vi "Wczytanie_ustawien_DI.vi"(8 "error in (no error)":errorcluster, 10 "Kanały cyfrowe in":refnum<vi>, 11 "Plik konf in":path) -> (0 "error out":errorcluster, 3 "Plik konf out":path)   [LabVIEW 2013]
doc: "Wczytuje ustawienia kontroli DI z pliku\nDI_Konfiguracja.txt"
uses:
  Kontrolki/GUI/DI_aktywacja.ctl
  Kontrolki/GUI/DI_prog.ctl
panel:
  out "output cluster":T1
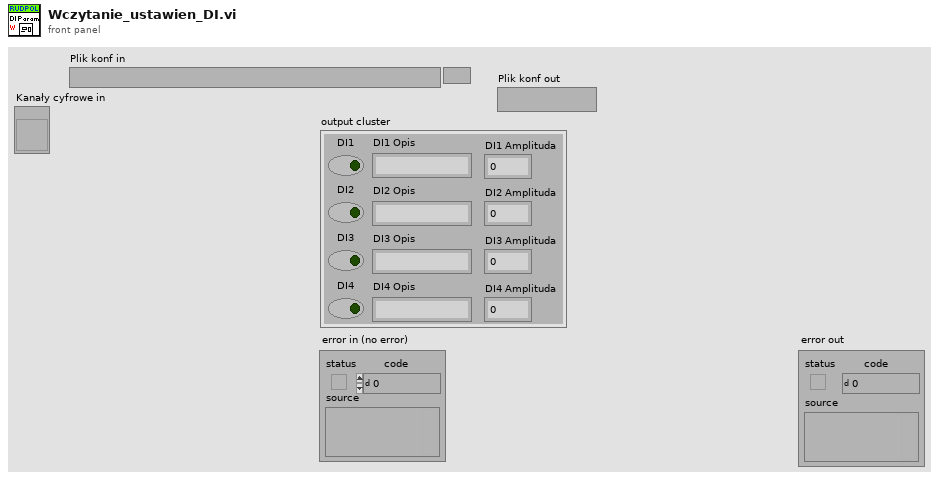
[diagram p1: front panel]
types:
  T1 = typedef "DI_aktywacja.ctl" = cluster{"DI1":bool, "DI2":bool, "DI3":bool, "DI4":bool, "DI1 Opis":string, "DI2 Opis":string, "DI3 Opis":string, "DI4 Opis":string, "DI1 Amplituda":dbl, "DI2 Amplituda":dbl, "DI3 Amplituda":dbl, "DI4 Amplituda":dbl}
  T2 = enum16{"open", "replace", "create", "open or create", "replace or create", "replace or create with confirmation"}
  T3 = typedef "DI_prog.ctl" = enum8{"2,5", "6,0", "12,0"}
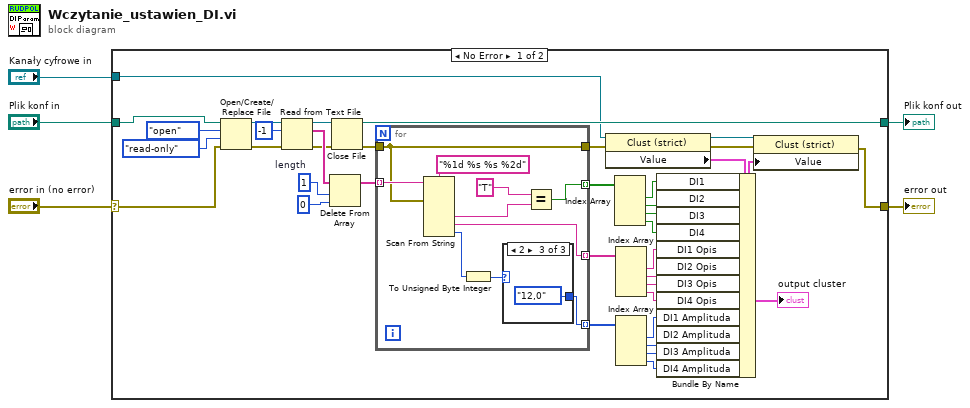
[diagram p0: block diagram]
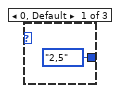
[diagram p2: hidden frame]
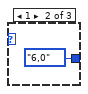
[diagram p3: hidden frame]
diagram:
  n1 = case shown="No Error" "error in (no error)" {
    selector: "error in (no error)" -> [w30 w57]
    tunnel: [w27 w57] -> w4
    tunnel: "Plik konf in" -> [w32 w56]
    tunnel: [w31 w56] -> w2
    tunnel: "Kanały cyfrowe in" -> [w23 _]
    frame No Error {
      w41 = 1  # length
      n2 = Open/Create/Replace File(file path (use dialog)=w32, error in=w30, operation (0:open)=T2."open", access (0:read/write)=enum16{"read/write", "read-only", "write-only"}."read-only") -> (refnum out=w36:refnum<file>, error out=w35:errorcluster)  [unwired: 2 in, 1 out]
      n3 = Read from Text File(file (use dialog)=w36, count=-1, error in=w35) -> (refnum out=w38:refnum<file>, text=w42:string[], error out=w37:errorcluster)  [unwired: 1 in, 1 out]
      n4 = Delete From Array(array=w42, length=w41, index=0) -> (array with subset deleted=w29:string[])  [unwired: 1 out]
      n5 = Close File(refnum=w38, error in=w37) -> (path=w31:path, error out=w28:errorcluster)
      n6 = for {
        tunnel: w29 -> [w51] mode=indexing
        tunnel: w28 -> [w50]
        tunnel: [w50] -> w24
        tunnel: [w47] -> w16 mode=indexing
        tunnel: [w46] -> w15 mode=indexing
        tunnel: [w45] -> w10 mode=indexing
        n7 = Scan From String(format string="%1d %s %s %2d", input string=w51, error in=w50) -> (output 2=w48:string, output 3=w46:string, output 4=w43:i32)  [unwired: 6 in, 3 out]
        n8 = To Unsigned Byte Integer(number=w43) -> (unsigned 8bit integer=w44:u8)
        n9 = case shown="2" w44 {
          tunnel: [DI_prog."2,5" ("DI1 Prog") DI_prog."6,0" ("DI1 Prog") DI_prog."12,0" ("DI1 Prog")] -> w45
          frame 0, Default {
          }
          frame 1 {
          }
          frame 2 {
          }
        }
        n10 = Equal?(x="T" ("y"), y=w48) -> (x = y?=w47:bool)
      }
      n11 = property class="Clust (strict)"(reference=w23, error in=w24) -> (reference out=w26:refnum<vi>, error out=w25:errorcluster, "Value"=w22:T1)
      n12 = Index Array(array=w16) -> (element #1=w20:bool, element #2=w19:bool, element #3=w18:bool, element #4=w17:bool)  [unwired: 4 in]
      n13 = Index Array(array=w15) -> (element #1=w14:string, element #2=w13:string, element #3=w12:string, element #4=w11:string)  [unwired: 4 in]
      n14 = Index Array(array=w10) -> (element #1=w9:T3, element #2=w8:T3, element #3=w7:T3, element #4=w6:T3)  [unwired: 4 in]
      n15 = Bundle By Name(cluster=w22, "DI1"=w20, "DI2"=w19, "DI3"=w18, "DI4"=w17, "DI1 Opis"=w14, "DI2 Opis"=w13, "DI3 Opis"=w12, "DI4 Opis"=w11, "DI1 Amplituda"=w9, "DI2 Amplituda"=w8, "DI3 Amplituda"=w7, "DI4 Amplituda"=w6) -> (w21:T1)
      "output cluster" <- w21
      n16 = property class="Clust (strict)"(reference=w26, error in=w25, "Value"=w21) -> (error out=w27:errorcluster)  [unwired: 1 out]
    }
    frame Error {
    }
  }
  "error out" <- w4
  "Plik konf out" <- w2
